vi "Read Preamble.vi"(8 "error in (no error)":errorcluster, 11 "Multipart Parser in":refnum<class "Multipart Parser.lvclass">) -> (0 "error out":errorcluster, 3 "Multipart Parser out":refnum<class "Multipart Parser.lvclass">)   [LabVIEW 2020, in "HTTP Utils.lvlib" / "Multipart Parser.lvclass"]
uses:
  Multipart Parser.lvclass
  Multipart Parser.lvclass/Multipart Parser.ctl
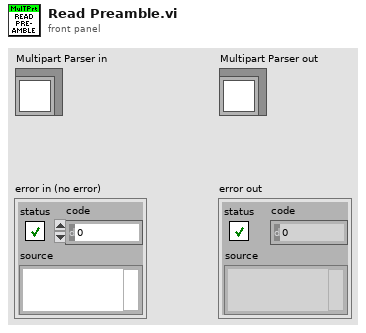
[diagram p1: front panel]
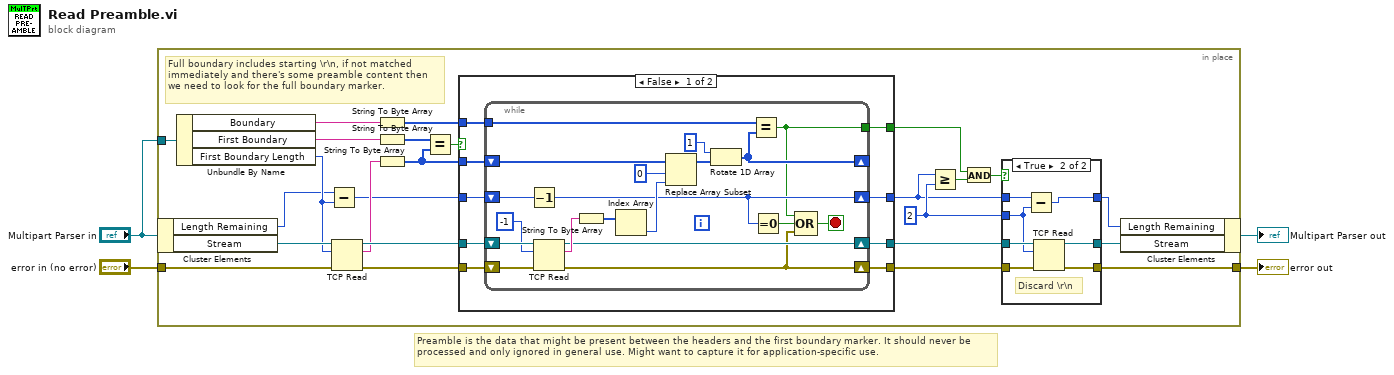
[diagram p0: block diagram]
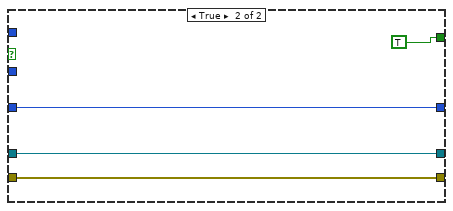
[diagram p2: hidden frame]
diagram:
  # "Preamble is the data that might be present between the headers and the first boundary marker. It should never be processed and only ignored in general use. Might want to capture it for application-specific use."
  n1 = in-place {
    in-place-border: "error in (no error)" -> [w27]
    in-place-border: "Multipart Parser in" -> [w29]
    in-place-border: [w8] -> w1
    w14 = u64 2 ("y")
    # "Full boundary includes starting \\r\\n, if not matched immediately and there's some preamble content then we need to look for the full boundary marker."
    n2 = in-place-cluster #1("Multipart Parser in") -> ("Length Remaining"=w20:u64, "Stream"=w28:refnum<k5>)
    n3 = Unbundle By Name(w29) -> ("Boundary"=w6:string, "First Boundary"=w24:string, "First Boundary Length"=w21:i32)
    n4 = Subtract(x=w20, y=w21) -> (x-y=w19:u64)
    n5 = TCP Read(connection ID=w28, bytes to read=w21, error in (no error)=w27) -> (connection ID out=w25:refnum<k5>, data out=w23:string, error out=w26:errorcluster)  [unwired: 2 in]
    n6 = String To Byte Array(string=w6) -> (unsigned byte array=w5:u8[])
    n7 = String To Byte Array(string=w24) -> (unsigned byte array=w18:u8[])
    n8 = String To Byte Array(string=w23) -> (unsigned byte array=w17:u8[])
    n9 = Equal?(x=w18, y=w17) -> (x = y?=w22:bool)
    n10 = case shown="False" w22 {
      tunnel: w26 -> [w38 w58]
      tunnel: w25 -> [w37 w59]
      tunnel: w19 -> [w36 w60]
      tunnel: w5 -> [w35 _]
      tunnel: w17 -> [w34 _]
      tunnel: [w33 w60] -> w13
      tunnel: [w32 TRUE] -> w12
      tunnel: [w31 w59] -> w11
      tunnel: [w30 w58] -> w10
      frame False {
        n11 = while {
          shift-right: [w40] -> w30
          shift-left: w38 -> [w56]
          shift-right: [w54] -> w31
          shift-left: w37 -> [w57]
          shift-right: [w42] -> w33
          shift-left: w36 -> [w44]
          tunnel: w35 -> [w46]
          shift-right: [w45] -> _
          shift-left: w34 -> [w52]
          tunnel: [w41] -> w32
          stop <- w53 stop-if-true
          n12 = Decrement(x=w44) -> (x-1=w42:u64)
          n13 = TCP Read(connection ID=w57, bytes to read=-1, error in (no error)=w56) -> (connection ID out=w54:refnum<k5>, data out=w55:string, error out=w40:errorcluster)  [unwired: 2 in]
          n14 = String To Byte Array(string=w55) -> (unsigned byte array=w50:u8[])
          n15 = Index Array(array=w50) -> (element=w49:u8)  [unwired: 1 in]
          n16 = Replace Array Subset(array=w52, new element=w49, index=0) -> (w48:u8[])
          n17 = Rotate 1D Array(1:w48, 2:1 ("n")) -> (0:w45:u8[])
          n18 = Equal?(x=w46, y=w45) -> (x = y?=w41:bool)
          n19 = Equal To 0?(x=w42) -> (x = 0?=w43:bool)
          n20 = Compound Arithmetic op=OR(w41, w43, w40) -> (w53:bool)
        }
      }
      frame True {
      }
    }
    n21 = Greater Or Equal?(x=w13, y=w14) -> (x >= y?=w16:bool)
    n22 = And(x=w12, y=w16) -> (x .and. y?=w15:bool)
    n23 = case shown="True" w15 {
      tunnel: w13 -> [w64 w71]
      tunnel: w11 -> [w63 w70]
      tunnel: w10 -> [w62 w69]
      tunnel: w14 -> [_ w68]
      tunnel: [w64 w65] -> w7
      tunnel: [w63 w66] -> w9
      tunnel: [w62 w67] -> w8
      frame False {
      }
      frame True {
        # "Discard \\r\\n"
        n24 = Subtract(x=w71, y=w68) -> (x-y=w65:u64)
        n25 = TCP Read(connection ID=w70, bytes to read=w68, error in (no error)=w69) -> (connection ID out=w66:refnum<k5>, error out=w67:errorcluster)  [unwired: 2 in, 1 out]
      }
    }
    n26 = in-place-cluster #1("Length Remaining"=w7, "Stream"=w9) -> (→"Multipart Parser out":refnum<class "Multipart Parser.lvclass">)
  }
  "error out" <- w1
